vi "genInterpretedIniFile.vi"(8 "error in":errorcluster, 11 "configuration file path":path) -> (0 "error out":errorcluster, 3 "interpretedIniFileContentArray":string[](array[string]))   [LabVIEW 2010]
uses:
  <vilib>/Utility/config.llb/Read Key (String).vi
  <vilib>/Utility/config.llb/NI_LVConfig.lvlib
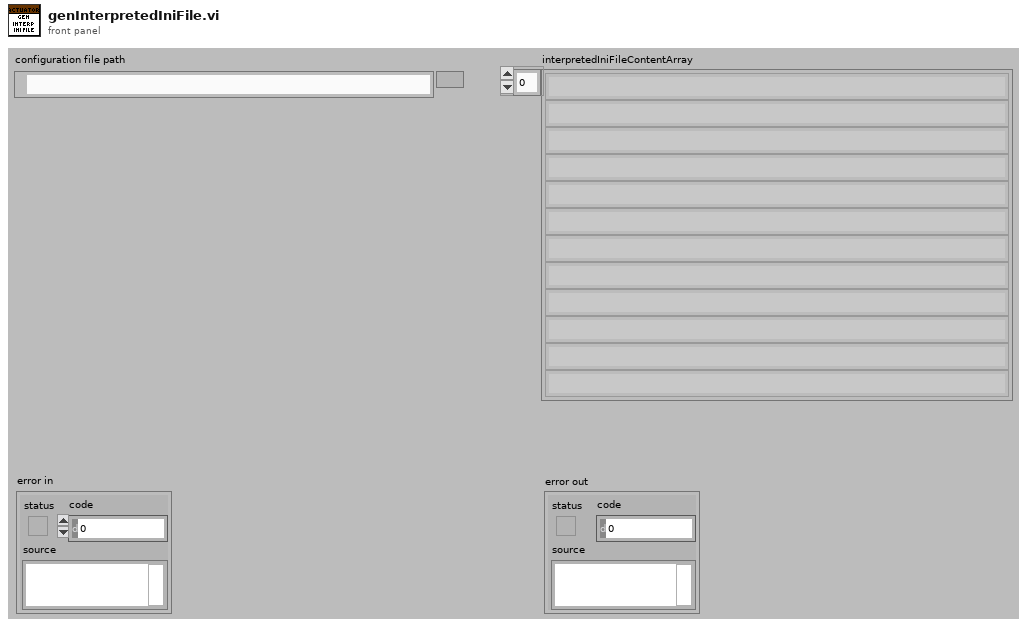
[diagram p1: front panel]
types:
  T1 = typedef "NI_LVConfig.lvlib/Config Data RefNum.ctl" = refnum<k1>
  T2 = enum16{"open", "replace", "create", "open or create", "replace or create", "replace or create with confirmation"}
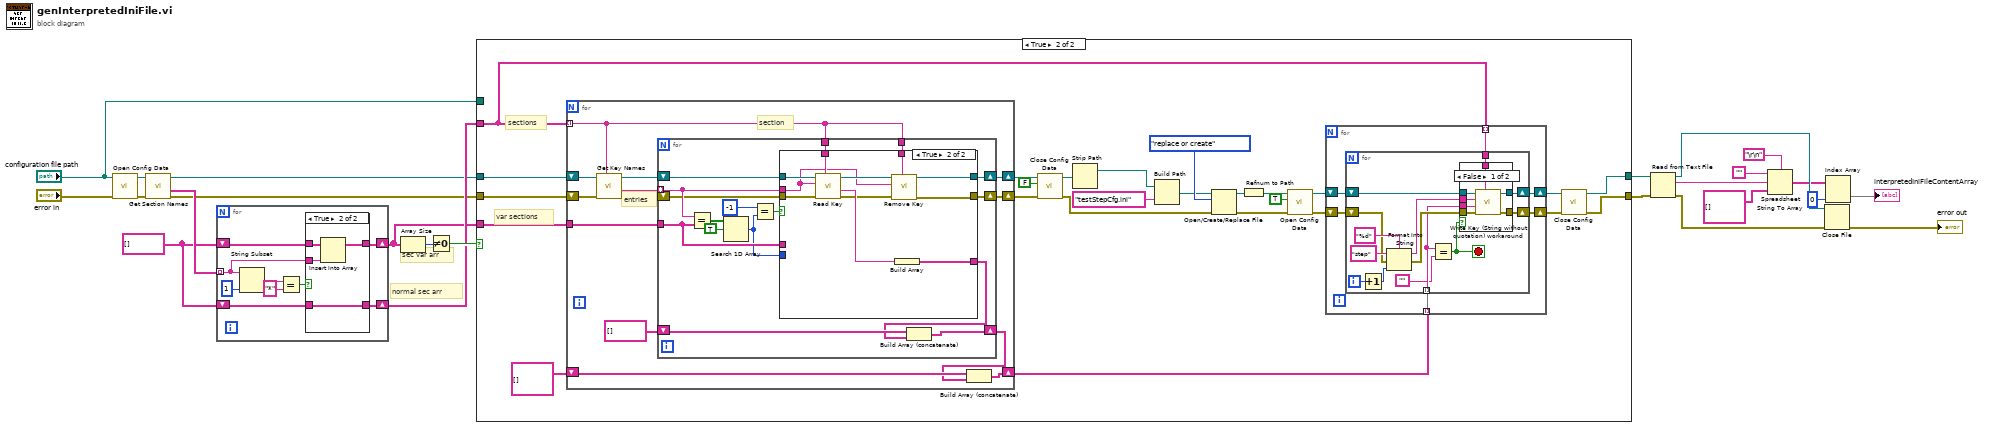
[diagram p0: block diagram]
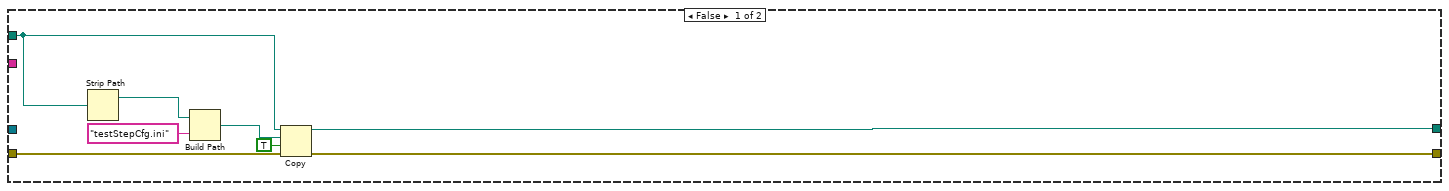
[diagram p2: hidden frame]
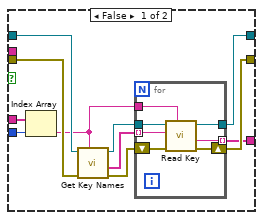
[diagram p4: hidden frame]
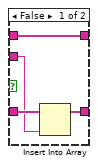
[diagram p5: hidden frame]
diagram:
  w19 = string[] []
  # "normal sec arr"
  # "sec var arr"
  n1 = call <vilib>:"Open Config Data.vi"("error in (no error)"="error in", "configuration file path"="configuration file path") -> ("error out"=w23:errorcluster, "refnum"=w24:T1)  [unwired: 7 in, 1 out]
  n2 = call <vilib>:"Get Section Names.vi"("error in (no error)"=w23, "refnum"=w24) -> ("error out"=w15:errorcluster, "section names"=w22:string[], "refnum out"=w4:T1)  [unwired: 7 in]
  n3 = for {
    tunnel: w22 -> [w29] mode=indexing
    shift-right: [w27] -> w16
    shift-left: w19 -> [w28]
    shift-right: [w25] -> w17
    shift-left: w19 -> [w26]
    n4 = String Subset(string=w29, length (rest)=1 ("length (rest)")) -> (substring=w32:string)  [unwired: 1 in]
    n5 = Equal?(x=w32, y="*") -> (x = y?=w30:bool)
    n6 = case shown="True" w30 {
      tunnel: w29 -> [w35 w41]
      tunnel: w28 -> [w37 w39]
      tunnel: [w37 w40] -> w27
      tunnel: w26 -> [w36 w38]
      tunnel: [w34 w38] -> w25
      frame False {
        n7 = Insert Into Array(array=w36, new element=w35) -> (w34:string[])  [unwired: 1 in]
      }
      frame True {
        n8 = Insert Into Array(array=w39, new element=w41) -> (w40:string[])  [unwired: 1 in]
      }
    }
  }
  n9 = Array Size(array=w16) -> (size(s)=w21:i32)
  n10 = Not Equal To 0?(x=w21) -> (x != 0?=w18:bool)
  n11 = case shown="True" w18 {
    tunnel: [w43 w71] -> w7
    tunnel: w16 -> [_ w70]
    tunnel: w17 -> [_ w68]
    tunnel: w15 -> [w47 w66]
    tunnel: "configuration file path" -> [w44 _]
    tunnel: [w42 w51] -> w6
    tunnel: w4 -> [_ w50]
    frame False {
      n12 = Strip Path(path=w44) -> (stripped path=w48:path)  [unwired: 1 out]
      n13 = Build Path(base path=w48, name or relative path="testStepCfg.ini" ("default name")) -> (appended path=w45:path)
      n14 = Copy(8:w47, 9:TRUE ("overwrite (F)"), 10:w45, 11:w44) -> (0:w43:errorcluster, 3:w42:path)  [unwired: 1 in, 1 out]
    }
    frame True {
      # "sections"
      # "var sections"
      n15 = for {
        tunnel: w68 -> [w104] mode=indexing
        shift-right: [w111] -> w73
        shift-left: w66 -> [w115]
        shift-right: [w112] -> w74
        shift-left: w50 -> [w116]
        tunnel: w70 -> [w109]
        shift-right: [w105] -> w67
        shift-left: string[][] [] -> [w107]
        # "entries"
        # "section"
        n16 = call <vilib>:"Get Key Names.vi"("section"=w104, "error in (no error)"=w115, "refnum"=w116) -> ("error out"=w114:errorcluster, "key names"=w110:string[], "refnum out"=w113:T1)  [unwired: 5 in, 1 out]
        n17 = for {
          tunnel: w110 -> [w126] mode=indexing
          tunnel: w104 -> [w128]
          shift-right: [w124] -> w111
          shift-left: w114 -> [w125]
          shift-right: [w123] -> w112
          shift-left: w113 -> [w127]
          tunnel: w109 -> [w122]
          shift-right: [w119] -> w106
          shift-left: string[] [] -> [w120]
          tunnel: w104 -> [w118]
          n18 = Equal?(x=w126, y=w122) -> (x = y?=w132:bool[])
          n19 = Search 1D Array(1D array=w132, element=TRUE) -> (index of element=w121:i32)  [unwired: 1 in]
          n20 = Equal?(x=-1, y=w121) -> (x = y?=w129:bool)
          n21 = case shown="True" w129 {
            tunnel: w128 -> [_ w161]
            tunnel: w127 -> [w141 w160]
            tunnel: w126 -> [_ w154]
            tunnel: w125 -> [w140 w159]
            tunnel: [w139 w152] -> w124
            tunnel: [w137 w151] -> w123
            tunnel: w122 -> [w143 _]
            tunnel: w121 -> [w142 _]
            tunnel: [w138 w157] -> w117
            tunnel: w118 -> [_ w153]
            frame False {
              n22 = Index Array(array=w143, index=w142) -> (element=w134:string)
              n23 = call <vilib>:"Get Key Names.vi"("section"=w134, "error in (no error)"=w140, "refnum"=w141) -> ("error out"=w133:errorcluster, "key names"=w135:string[], "refnum out"=w136:T1)  [unwired: 5 in, 1 out]
              n24 = for {
                tunnel: w134 -> [w150]
                tunnel: w136 -> [w149]
                tunnel: w135 -> [w148] mode=indexing
                shift-right: [w146] -> w139
                shift-left: w133 -> [w147]
                tunnel: [w145] -> w138 mode=indexing
                tunnel: [w144] -> w137
                n25 = call-poly <vilib>:"Read Key.vi"("section"=w150, "error in (no error)"=w147, "key"=w148, "refnum"=w149) -> ("error out"=w146:errorcluster, "value"=w145:string, "refnum out"=w144:T1)  [unwired: 4 in, 1 out]
              }
            }
            frame True {
              n26 = call-poly <vilib>:"Read Key.vi"("section"=w161, "error in (no error)"=w159, "key"=w154, "refnum"=w160) -> ("error out"=w155:errorcluster, "value"=w158:string, "refnum out"=w156:T1)  [unwired: 4 in, 1 out]
              n27 = call <vilib>:"Remove Key.vi"("section"=w153, "error in (no error)"=w155, "key"=w154, "refnum"=w156) -> ("error out"=w152:errorcluster, "refnum out"=w151:T1)  [unwired: 5 in, 1 out]
              n28 = Build Array(w158) -> (w157:string[])
            }
          }
          n29 = Build Array (concatenate)(w120, w117) -> (w119:string[])
        }
        n30 = Build Array (concatenate)(w107, w106) -> (w105:string[][])
      }
      n31 = call <vilib>:"Close Config Data.vi"("error in (no error)"=w73, "write file if changed (T)"=FALSE, "refnum"=w74) -> ("error out"=w52:errorcluster, "file path"=w54:path)  [unwired: 7 in]
      n32 = Strip Path(path=w54) -> (stripped path=w55:path)  [unwired: 1 out]
      n33 = Build Path(base path=w55, name or relative path="testStepCfg.ini" ("default name")) -> (appended path=w53:path)
      n34 = Open/Create/Replace File(file path (use dialog)=w53, error in=w52, operation (0:open)=T2."replace or create") -> (refnum out=w60:refnum<file>, error out=w58:errorcluster)  [unwired: 3 in, 1 out]
      n35 = Refnum to Path(1:w60) -> (0:w59:path)
      n36 = call <vilib>:"Open Config Data.vi"("error in (no error)"=w58, "create file if necessary (T)"=TRUE, "configuration file path"=w59) -> ("error out"=w63:errorcluster, "refnum"=w64:T1)  [unwired: 6 in, 1 out]
      n37 = for {
        tunnel: w68 -> [w75] mode=indexing
        shift-right: [w79] -> w61
        shift-left: w64 -> [w80]
        shift-right: [w77] -> w62
        shift-left: w63 -> [w78]
        tunnel: w67 -> [w76] mode=indexing
        n38 = for {
          shift-right: [w93] -> w79
          shift-left: w80 -> [w94]
          shift-right: [w92] -> w77
          shift-left: w78 -> [w89]
          tunnel: w76 -> [w84] mode=indexing
          tunnel: w75 -> [w81]
          i -> [w86]
          stop <- w82 stop-if-true
          n39 = Increment(x=w86) -> (x+1=w85:i32)
          n40 = Format Into String(format string="%d", initial string="step", error in=w89, w85) -> (resulting string=w87:string, error out=w88:errorcluster)
          n41 = Equal?(x=w84, y="") -> (x = y?=w82:bool)
          n42 = case shown="False" w82 {
            tunnel: w94 -> [w101 w103]
            tunnel: [w96 w103] -> w93
            tunnel: [w97 w102] -> w92
            tunnel: w88 -> [w98 w102]
            tunnel: w87 -> [w100 _]
            tunnel: w84 -> [w99 _]
            tunnel: w81 -> [w95 _]
            frame False {
              n43 = call <vilib>:"Write Key (String without quotation) workaround.vi"("section"=w95, "error in (no error)"=w98, "value"=w99, "key"=w100, "refnum"=w101) -> ("error out"=w97:errorcluster, "refnum out"=w96:T1)  [unwired: 4 in, 1 out]
            }
            frame True {
            }
          }
        }
      }
      n44 = call <vilib>:"Close Config Data.vi"("error in (no error)"=w62, "refnum"=w61) -> ("error out"=w71:errorcluster, "file path"=w51:path)  [unwired: 8 in]
    }
  }
  n45 = Read from Text File(file (use dialog)=w6, error in=w7) -> (refnum out=w13:refnum<file>, text=w8:string, error out=w12:errorcluster)  [unwired: 2 in, 1 out]
  n46 = Spreadsheet String To Array(delimiter (Tab)="\r\n", format string="", spreadsheet string=w8, array type (2D Dbl)=string[][] []) -> (array=w3:string[][])
  n47 = Close File(refnum=w13, error in=w12) -> (error out=→"error out":errorcluster)  [unwired: 1 out]
  n48 = Index Array(array=w3, index (col)=0 ("disabled index (col)")) -> (element=→"interpretedIniFileContentArray":string[])  [unwired: 1 in]
